vi "Init.vi"(8 "error in (no error)":errorcluster, 9 "Trigger Configuration In":variant, 10 "DIO Configuration In":variant, 11 "NIDIO in":refnum<class "NIDIO.lvclass">) -> (0 "error out":errorcluster, 3 "NIDIO out":refnum<class "NIDIO.lvclass">)   [LabVIEW 2015, in "NIDIO.lvclass"]
uses:
  NIDIO.lvclass
  NIDIO.lvclass/NIDIO.ctl
  <vilib>/DAQmx/create/channels.llb/DAQmx Create Channel (DO-Digital Output).vi
  DIO.lvclass
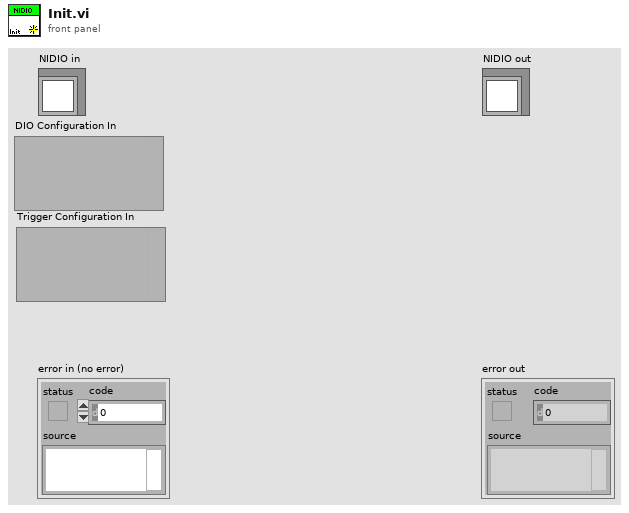
[diagram p1: front panel]
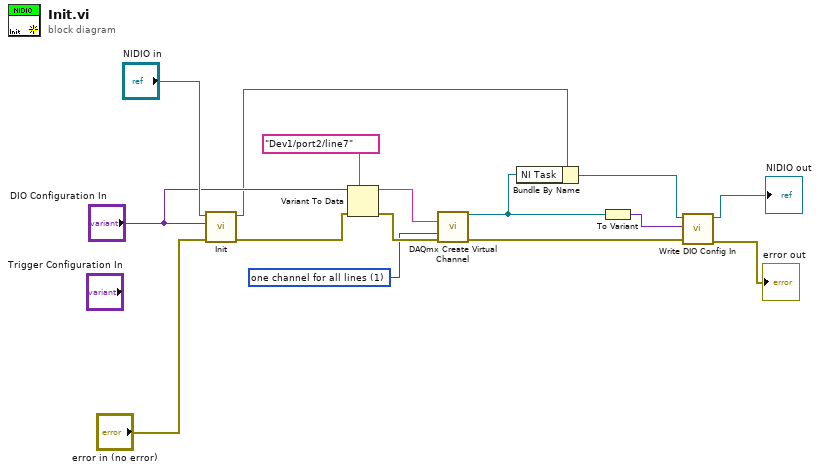
[diagram p0: block diagram]
diagram:
  w5 = 1 items=["one channel for each line", "one channel for all lines"] ("line grouping")
  n1 = call-parent "Init.vi"("error in (no error)"="error in (no error)", "DIO Config In"="DIO Configuration In", "DIO in"="NIDIO in") -> ("error out"=w11:errorcluster, "DIO out"=w3:refnum<class "NIDIO.lvclass">)  [unwired: 7 in]
  n2 = Variant To Data(error in=w11, type=tag "Dev1/port2/line7" ("lines"), Variant="DIO Configuration In") -> (data=w6:tag, error out=w12:errorcluster)
  n3 = call-poly <vilib>:"DAQmx Create Virtual Channel.vi"("lines"=w6, "line grouping"=w5, "error in"=w12) -> ("task out"=w4:refnum<k21>, "error out"=w1:errorcluster)  [unwired: 11 in]
  n4 = Bundle By Name(cluster=w3, "NI Task"=w4) -> (w2:refnum<class "NIDIO.lvclass">)
  n5 = To Variant(anything=w4) -> (Variant=w10:variant)
  n6 = call-dynamic "Write DIO Config In.vi"("error in (no error)"=w1, "DIO Config In"=w10, "DIO in"=w2) -> ("error out"=→"error out":errorcluster, "DIO out"=→"NIDIO out":refnum<class "NIDIO.lvclass">)  [unwired: 7 in]
